vi "NetA_RSZVL_MatchIDNStr.vi"(8 "error in":errorcluster, 10 "IDNStr":string) -> (0 "error out":errorcluster, 2 "IDN match":bool, 3 "ClassLibraryFile":path)   [LabVIEW 2014]
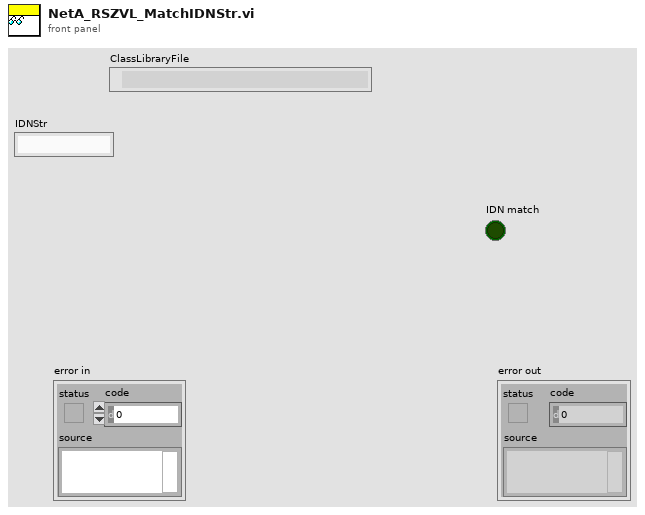
[diagram p1: front panel]
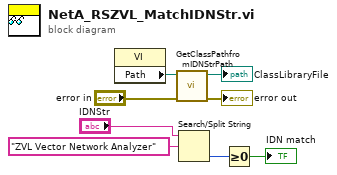
[diagram p0: block diagram]
diagram:
  n1 = property class="VI"() -> ("Path"=w8:path)  [unwired: 2 in, 2 out]
  n2 = call "GetClassPathfromIDNStrPath.vi"("error in (no error)"="error in", "Path in"=w8) -> ("error out"=→"error out":errorcluster, "Path out"=→"ClassLibraryFile":path)  [unwired: 8 in]
  n3 = Search/Split String(string="IDNStr", search string/char (-)="ZVL Vector Network Analyzer") -> (offset of match=w3:i32)  [unwired: 1 in, 2 out]
  n4 = Greater Or Equal To 0?(x=w3) -> (x >= 0?=→"IDN match":bool)
